vi "Facade 1.vi"(0 "Data In":T4=["ListboxMeasurementMeth", "ListboxMeasurementTechnique", "ListboxMeasurementArea", "ListboxCpr", "HospitalName", "HospitalAddress"], 2 "Display State In":T2, 3 "Container State":T3) -> (6 "Data Out":T4=["ListboxMeasurementMeth", "ListboxMeasurementTechnique", "ListboxMeasurementArea", "ListboxCpr", "HospitalName", "HospitalAddress"], 7 "Display State Out":T2, 8 "Action":T1)   [LabVIEW 2013, in "main.lvlib" / "XControl 1.xctl"]
uses:
  XControl 1.xctl
  Data 1.ctl
  <vilib>/_xctls/Container State.ctl
  State 1.ctl
  <vilib>/_xctls/Action.ctl
  <vilib>/_xctls/XControlSupport.lvlib
panel:
  # "1. Drop the controls that make up the appearance\nof the XControl here.\n\n2. Resize the window to fit the controls\n\n3. If the XControl is of fixed size,  make the \n window not resizable from VI Properties->Window Appearance.\n\n4. If you want the controls to automatically size when the XControl sizes, check  \"Scale all objects on front panel when window resizes\" in File->VI Properties->Window Size page.\n\n5. Show the block diagram and handle events for the controls on this panel."
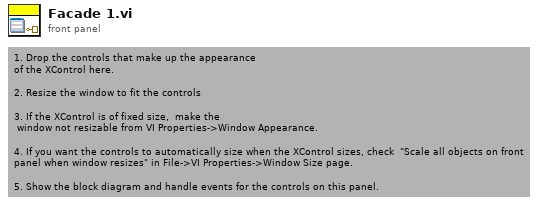
[diagram p1: front panel]
types:
  T1 = typedef "XControlSupport.lvlib/Action.ctl" = cluster{"Data Changed?":bool, "State Changed?":bool, "Action Name":string}
  T2 = typedef "main.lvlib/XControl 1.xctl/State 1.ctl" = cluster{"Numeric":dbl}
  T3 = typedef "XControlSupport.lvlib/Container State.ctl" = cluster{"Indicator?":bool, "Run Mode?":bool, " Refnum":refnum<vi>}
  T4 = typedef "main.lvlib/XControl 1.xctl/Data 1.ctl" = string[]
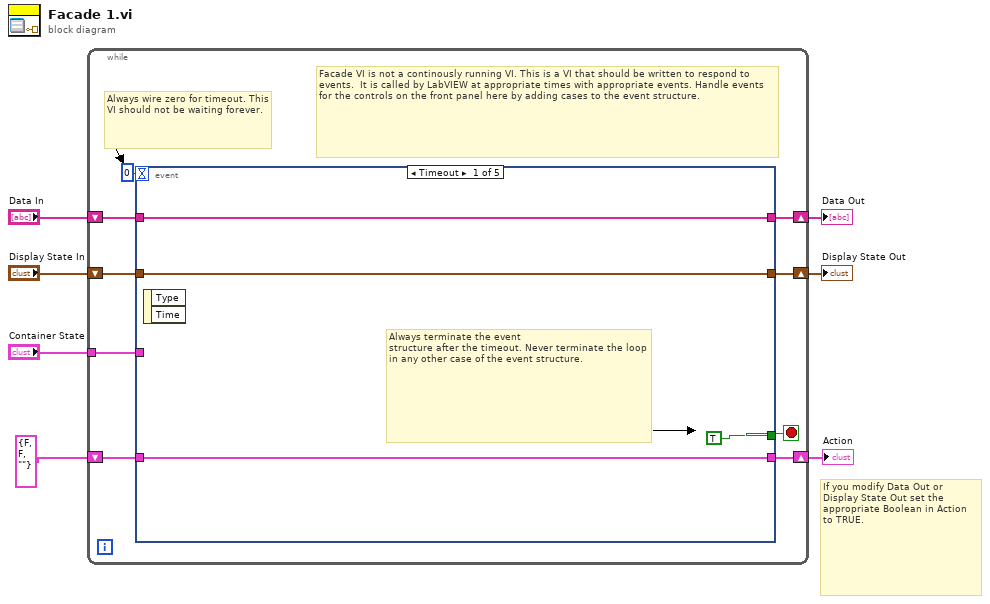
[diagram p0: block diagram]
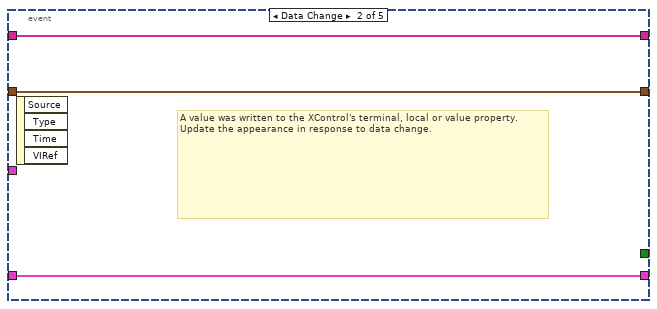
[diagram p2: hidden frame]
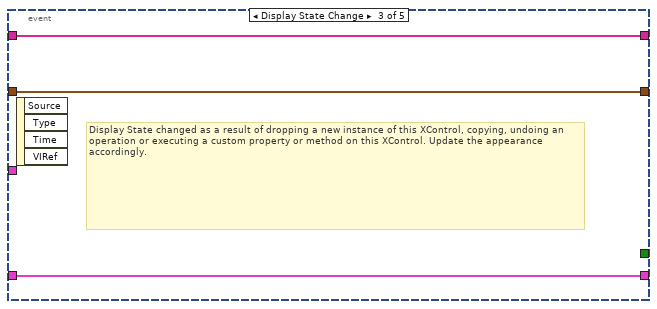
[diagram p3: hidden frame]
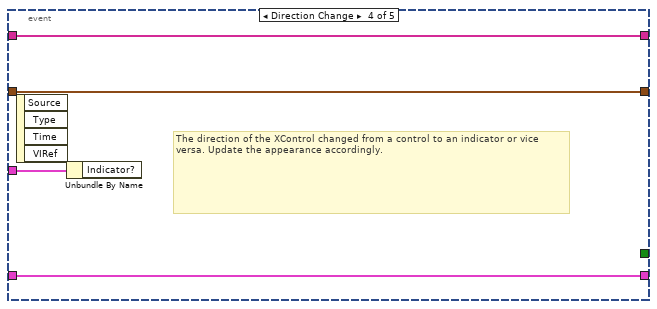
[diagram p4: hidden frame]
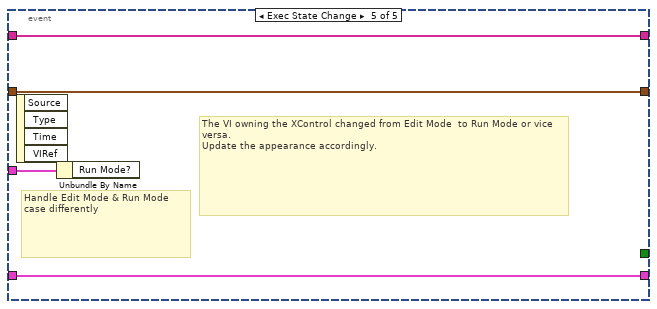
[diagram p5: hidden frame]
diagram:
  # "If you modify Data Out or\nDisplay State Out set the\nappropriate Boolean in Action\nto TRUE."
  n1 = while {
    shift-right: [w15] -> w4
    shift-left: "Display State In" -> [w16]
    tunnel: "Container State" -> [w12]
    shift-right: [w10] -> w7
    shift-left: "Data In" -> [w11]
    shift-right: [w8] -> w2
    shift-left: T1 {"Data Changed?"=FALSE, "State Changed?"=FALSE, "Action Name"=""} ("Action") -> [w9]
    stop <- w14 stop-if-true
    # "Facade VI is not a continously running VI. This is a VI that should be written to respond to events.  It is called by LabVIEW at appropriate times with appropriate events. Handle events for the controls on the front panel here by adding cases to the event structure."
    # "Always wire zero for timeout. This\nVI should not be waiting forever."
    n2 = event shown="[0] Timeout" {
      selector: _ -> [_ _ _ _ _]
      dyn-events: _ -> [_ _ _ _ _]
      timeout: 0 -> [_ _ _ _ _]
      tunnel: w16 -> [w18 w22 w26 w29 w33]
      tunnel: [w18 w22 w26 w29 w33] -> w15
      tunnel: [TRUE _ _ _ _] -> w14
      tunnel: w12 -> [_ _ _ w30 w34]
      tunnel: w11 -> [w17 w23 w25 w28 w32]
      tunnel: [w17 w23 w25 w28 w32] -> w10
      tunnel: [w19 w21 w24 w27 w31] -> w8
      tunnel: w9 -> [w19 w21 w24 w27 w31]
      event Timeout {
        # "Always terminate the event\nstructure after the timeout. Never terminate the loop in any other case of the event structure."
        n3 = event-data() -> ()  [unwired: 1 in, 2 out]
      }
      event Data Change {
        # "A value was written to the XControl's terminal, local or value property.\nUpdate the appearance in response to data change."
        n4 = event-data() -> ()  [unwired: 1 in, 4 out]
      }
      event Display State Change {
        # "Display State changed as a result of dropping a new instance of this XControl, copying, undoing an operation or executing a custom property or method on this XControl. Update the appearance accordingly."
        n5 = event-data() -> ()  [unwired: 1 in, 4 out]
      }
      event Direction Change {
        # "The direction of the XControl changed from a control to an indicator or vice versa. Update the appearance accordingly."
        n6 = event-data() -> ()  [unwired: 1 in, 4 out]
        n7 = Unbundle By Name(w30) -> ()  [unwired: 1 out]
      }
      event Exec State Change {
        # "The VI owning the XControl changed from Edit Mode  to Run Mode or vice versa.\nUpdate the appearance accordingly."
        # "Handle Edit Mode & Run Mode\ncase differently"
        n8 = event-data() -> ()  [unwired: 1 in, 4 out]
        n9 = Unbundle By Name(w34) -> ()  [unwired: 1 out]
      }
    }
  }
  "Display State Out" <- w4
  "Data Out" <- w7
  "Action" <- w2
